vi "ParseSpeeds.vi"(8 "inputCluster":T1={"swerveModules"={"leftFront"={"driveCANID"=0.0, "angleCANID"=0, "canCoderCANID"=0.0, "moduleName"="", "driveMotorNeutralMode"=enum."EEPROMSetting", "driveCurrentLimitConfig"={"Enable?"=FALSE, "Current Limit"=0.0, "Threshold Current"=0.0, "Threshold Time"=0.0}, "driveFeedbackDevice"=0, "driveInitialSensorPosition"=0.0, "driveEnableVoltageComp"=FALSE, "driveVoltageComp"=0.0, "driveRampRate"=0.0, "angleCurrentLimit"=0.0, "angleSensorType"=enum."No Sensor", "angleMotorType"=enum."Brushed", "angleConversionFactor"=0.0, "anglePIDRamp"=0.0, "angleVoltageComp"=0.0, "angleIdleMode"=enum."Coast", "cancoderConfig"={"Sensor Initialization Strategy"=enum."Boot To Zero", "Absolute Sensor Range"=enum."Unsigned [0 to 360)", "Velocity Measurement Period"=0, "Velocity Measurement Window"=0, "Magnet Offset (Degrees)"=0.0, "Sensor Direction"=FALSE, "Sensor Coefficient"=0.0, "Unit String"="", "Sensor Time Base"=enum."Per100Ms_Legacy"}, "angleInitialSensorPosition"=0.0}, "rightFront"={"driveCANID"=0.0, "angleCANID"=0, "canCoderCANID"=0.0, "moduleName"="", "driveMotorNeutralMode"=enum."EEPROMSetting", "driveCurrentLimitConfig"={"Enable?"=FALSE, "Current Limit"=0.0, "Threshold Current"=0.0, "Threshold Time"=0.0}, "driveFeedbackDevice"=0, "driveInitialSensorPosition"=0.0, "driveEnableVoltageComp"=FALSE, "driveVoltageComp"=0.0, "driveRampRate"=0.0, "angleCurrentLimit"=0.0, "angleSensorType"=enum."No Sensor", "angleMotorType"=enum."Brushed", "angleConversionFactor"=0.0, "anglePIDRamp"=0.0, "angleVoltageComp"=0.0, "angleIdleMode"=enum."Coast", "cancoderConfig"={"Sensor Initialization Strategy"=enum."Boot To Zero", "Absolute Sensor Range"=enum."Unsigned [0 to 360)", "Velocity Measurement Period"=0, "Velocity Measurement Window"=0, "Magnet Offset (Degrees)"=0.0, "Sensor Direction"=FALSE, "Sensor Coefficient"=0.0, "Unit String"="", "Sensor Time Base"=enum."Per100Ms_Legacy"}, "angleInitialSensorPosition"=0.0}, "leftRear"={"driveCANID"=0.0, "angleCANID"=0, "canCoderCANID"=0.0, "moduleName"="", "driveMotorNeutralMode"=enum."EEPROMSetting", "driveCurrentLimitConfig"={"Enable?"=FALSE, "Current Limit"=0.0, "Threshold Current"=0.0, "Threshold Time"=0.0}, "driveFeedbackDevice"=0, "driveInitialSensorPosition"=0.0, "driveEnableVoltageComp"=FALSE, "driveVoltageComp"=0.0, "driveRampRate"=0.0, "angleCurrentLimit"=0.0, "angleSensorType"=enum."No Sensor", "angleMotorType"=enum."Brushed", "angleConversionFactor"=0.0, "anglePIDRamp"=0.0, "angleVoltageComp"=0.0, "angleIdleMode"=enum."Coast", "cancoderConfig"={"Sensor Initialization Strategy"=enum."Boot To Zero", "Absolute Sensor Range"=enum."Unsigned [0 to 360)", "Velocity Measurement Period"=0, "Velocity Measurement Window"=0, "Magnet Offset (Degrees)"=0.0, "Sensor Direction"=FALSE, "Sensor Coefficient"=0.0, "Unit String"="", "Sensor Time Base"=enum."Per100Ms_Legacy"}, "angleInitialSensorPosition"=0.0}, "rightRear"={"driveCANID"=0.0, "angleCANID"=0, "canCoderCANID"=0.0, "moduleName"="", "driveMotorNeutralMode"=enum."EEPROMSetting", "driveCurrentLimitConfig"={"Enable?"=FALSE, "Current Limit"=0.0, "Threshold Current"=0.0, "Threshold Time"=0.0}, "driveFeedbackDevice"=0, "driveInitialSensorPosition"=0.0, "driveEnableVoltageComp"=FALSE, "driveVoltageComp"=0.0, "driveRampRate"=0.0, "angleCurrentLimit"=0.0, "angleSensorType"=enum."No Sensor", "angleMotorType"=enum."Brushed", "angleConversionFactor"=0.0, "anglePIDRamp"=0.0, "angleVoltageComp"=0.0, "angleIdleMode"=enum."Coast", "cancoderConfig"={"Sensor Initialization Strategy"=enum."Boot To Zero", "Absolute Sensor Range"=enum."Unsigned [0 to 360)", "Velocity Measurement Period"=0, "Velocity Measurement Window"=0, "Magnet Offset (Degrees)"=0.0, "Sensor Direction"=FALSE, "Sensor Coefficient"=0.0, "Unit String"="", "Sensor Time Base"=enum."Per100Ms_Legacy"}, "angleInitialSensorPosition"=0.0}}, "offsets"={"leftFrontAngleOffset"=-143.789, "leftRearAngleOffset"=-94.834, "rightFrontAngleOffset"=55.1074, "rightRearAngleOffset"=42.8906}, "limits"={"maxVelocity"=0.0, "maxOverdriveVelocity"=0.0, "maxAcceleration"=0.0, "maxPickupVelocity"=0.0}, "speeds"={"intakeSuckSpeed"=0.0, "intakeSpitSpeed"=0.0, "indexerSuckSpeed"=0.0, "indexerSpitSpeed"=0.0, "indexerShootSpeed"=0.0, "indexerBumpBackSpeed"=0.0, "shooterSpinupSpeed"=0.0, "kickupSpinupSpeed"=0.0, "shooterLowShootSpeed"=0.0, "shooterHighShootSpeed"=0.0}, "positions"={"intakeStarting"=0.0, "intakeStow"=0.0, "intakeSuck"=0.0, "armPounce"=0.0, "armStow"=0.0, "armUp"=0.0, "winchPounce"=0.0, "winchOut"=0.0, "winchStow"=0.0, "intakeSpit"=0.0, "winchBarEngage"=0.0, "winchBottomClimb"=0.0, "hoodHighShoot"=0.0}, "inversions"={"rightShooter"=FALSE, "leftShooter"=FALSE}} {"swerveModules"."rightRear"."cancoderConfig"."Velocity Measurement Period" items=["Period_1ms"=1, "Period_2ms"=2, "Period_5ms"=5, "Period_10ms"=10, "Period_20ms"=20, "Period_25ms"=25, "Period_50ms"=50, "Period_100ms"=100]; "swerveModules"."rightRear"."cancoderConfig"."Sensor Coefficient" format="%#_9g"; "swerveModules"."rightRear"."driveFeedbackDevice" items=["Integrated Sensor"=1, "Sensor Sum (S0 + S1)"=9, "Sensor Difference (D0 - D1)"=10, "Remote Source 0"=11, "Remote Source 1"=12, "None"=14, "Software Emulated"=15]; "swerveModules"."leftRear"."cancoderConfig"."Velocity Measurement Period" items=["Period_1ms"=1, "Period_2ms"=2, "Period_5ms"=5, "Period_10ms"=10, "Period_20ms"=20, "Period_25ms"=25, "Period_50ms"=50, "Period_100ms"=100]; "swerveModules"."leftRear"."cancoderConfig"."Sensor Coefficient" format="%#_9g"; "swerveModules"."leftRear"."driveFeedbackDevice" items=["Integrated Sensor"=1, "Sensor Sum (S0 + S1)"=9, "Sensor Difference (D0 - D1)"=10, "Remote Source 0"=11, "Remote Source 1"=12, "None"=14, "Software Emulated"=15]; "swerveModules"."rightFront"."cancoderConfig"."Velocity Measurement Period" items=["Period_1ms"=1, "Period_2ms"=2, "Period_5ms"=5, "Period_10ms"=10, "Period_20ms"=20, "Period_25ms"=25, "Period_50ms"=50, "Period_100ms"=100]; "swerveModules"."rightFront"."cancoderConfig"."Sensor Coefficient" format="%#_9g"; "swerveModules"."rightFront"."driveFeedbackDevice" items=["Integrated Sensor"=1, "Sensor Sum (S0 + S1)"=9, "Sensor Difference (D0 - D1)"=10, "Remote Source 0"=11, "Remote Source 1"=12, "None"=14, "Software Emulated"=15]; "swerveModules"."leftFront"."cancoderConfig"."Velocity Measurement Period" items=["Period_1ms"=1, "Period_2ms"=2, "Period_5ms"=5, "Period_10ms"=10, "Period_20ms"=20, "Period_25ms"=25, "Period_50ms"=50, "Period_100ms"=100]; "swerveModules"."leftFront"."cancoderConfig"."Sensor Coefficient" format="%#_9g"; "swerveModules"."leftFront"."driveFeedbackDevice" items=["Integrated Sensor"=1, "Sensor Sum (S0 + S1)"=9, "Sensor Difference (D0 - D1)"=10, "Remote Source 0"=11, "Remote Source 1"=12, "None"=14, "Software Emulated"=15]}, 9 "configRef":T14) -> (2 "outputCluster":T1={"swerveModules"={"leftFront"={"driveCANID"=0.0, "angleCANID"=0, "canCoderCANID"=0.0, "moduleName"="", "driveMotorNeutralMode"=enum."EEPROMSetting", "driveCurrentLimitConfig"={"Enable?"=FALSE, "Current Limit"=0.0, "Threshold Current"=0.0, "Threshold Time"=0.0}, "driveFeedbackDevice"=0, "driveInitialSensorPosition"=0.0, "driveEnableVoltageComp"=FALSE, "driveVoltageComp"=0.0, "driveRampRate"=0.0, "angleCurrentLimit"=0.0, "angleSensorType"=enum."No Sensor", "angleMotorType"=enum."Brushed", "angleConversionFactor"=0.0, "anglePIDRamp"=0.0, "angleVoltageComp"=0.0, "angleIdleMode"=enum."Coast", "cancoderConfig"={"Sensor Initialization Strategy"=enum."Boot To Zero", "Absolute Sensor Range"=enum."Unsigned [0 to 360)", "Velocity Measurement Period"=0, "Velocity Measurement Window"=0, "Magnet Offset (Degrees)"=0.0, "Sensor Direction"=FALSE, "Sensor Coefficient"=0.0, "Unit String"="", "Sensor Time Base"=enum."Per100Ms_Legacy"}, "angleInitialSensorPosition"=0.0}, "rightFront"={"driveCANID"=0.0, "angleCANID"=0, "canCoderCANID"=0.0, "moduleName"="", "driveMotorNeutralMode"=enum."EEPROMSetting", "driveCurrentLimitConfig"={"Enable?"=FALSE, "Current Limit"=0.0, "Threshold Current"=0.0, "Threshold Time"=0.0}, "driveFeedbackDevice"=0, "driveInitialSensorPosition"=0.0, "driveEnableVoltageComp"=FALSE, "driveVoltageComp"=0.0, "driveRampRate"=0.0, "angleCurrentLimit"=0.0, "angleSensorType"=enum."No Sensor", "angleMotorType"=enum."Brushed", "angleConversionFactor"=0.0, "anglePIDRamp"=0.0, "angleVoltageComp"=0.0, "angleIdleMode"=enum."Coast", "cancoderConfig"={"Sensor Initialization Strategy"=enum."Boot To Zero", "Absolute Sensor Range"=enum."Unsigned [0 to 360)", "Velocity Measurement Period"=0, "Velocity Measurement Window"=0, "Magnet Offset (Degrees)"=0.0, "Sensor Direction"=FALSE, "Sensor Coefficient"=0.0, "Unit String"="", "Sensor Time Base"=enum."Per100Ms_Legacy"}, "angleInitialSensorPosition"=0.0}, "leftRear"={"driveCANID"=0.0, "angleCANID"=0, "canCoderCANID"=0.0, "moduleName"="", "driveMotorNeutralMode"=enum."EEPROMSetting", "driveCurrentLimitConfig"={"Enable?"=FALSE, "Current Limit"=0.0, "Threshold Current"=0.0, "Threshold Time"=0.0}, "driveFeedbackDevice"=0, "driveInitialSensorPosition"=0.0, "driveEnableVoltageComp"=FALSE, "driveVoltageComp"=0.0, "driveRampRate"=0.0, "angleCurrentLimit"=0.0, "angleSensorType"=enum."No Sensor", "angleMotorType"=enum."Brushed", "angleConversionFactor"=0.0, "anglePIDRamp"=0.0, "angleVoltageComp"=0.0, "angleIdleMode"=enum."Coast", "cancoderConfig"={"Sensor Initialization Strategy"=enum."Boot To Zero", "Absolute Sensor Range"=enum."Unsigned [0 to 360)", "Velocity Measurement Period"=0, "Velocity Measurement Window"=0, "Magnet Offset (Degrees)"=0.0, "Sensor Direction"=FALSE, "Sensor Coefficient"=0.0, "Unit String"="", "Sensor Time Base"=enum."Per100Ms_Legacy"}, "angleInitialSensorPosition"=0.0}, "rightRear"={"driveCANID"=0.0, "angleCANID"=0, "canCoderCANID"=0.0, "moduleName"="", "driveMotorNeutralMode"=enum."EEPROMSetting", "driveCurrentLimitConfig"={"Enable?"=FALSE, "Current Limit"=0.0, "Threshold Current"=0.0, "Threshold Time"=0.0}, "driveFeedbackDevice"=0, "driveInitialSensorPosition"=0.0, "driveEnableVoltageComp"=FALSE, "driveVoltageComp"=0.0, "driveRampRate"=0.0, "angleCurrentLimit"=0.0, "angleSensorType"=enum."No Sensor", "angleMotorType"=enum."Brushed", "angleConversionFactor"=0.0, "anglePIDRamp"=0.0, "angleVoltageComp"=0.0, "angleIdleMode"=enum."Coast", "cancoderConfig"={"Sensor Initialization Strategy"=enum."Boot To Zero", "Absolute Sensor Range"=enum."Unsigned [0 to 360)", "Velocity Measurement Period"=0, "Velocity Measurement Window"=0, "Magnet Offset (Degrees)"=0.0, "Sensor Direction"=FALSE, "Sensor Coefficient"=0.0, "Unit String"="", "Sensor Time Base"=enum."Per100Ms_Legacy"}, "angleInitialSensorPosition"=0.0}}, "offsets"={"leftFrontAngleOffset"=-143.789, "leftRearAngleOffset"=-94.834, "rightFrontAngleOffset"=55.1074, "rightRearAngleOffset"=42.8906}, "limits"={"maxVelocity"=0.0, "maxOverdriveVelocity"=0.0, "maxAcceleration"=0.0, "maxPickupVelocity"=0.0}, "speeds"={"intakeSuckSpeed"=0.0, "intakeSpitSpeed"=0.0, "indexerSuckSpeed"=0.0, "indexerSpitSpeed"=0.0, "indexerShootSpeed"=0.0, "indexerBumpBackSpeed"=0.0, "shooterSpinupSpeed"=0.0, "kickupSpinupSpeed"=0.0, "shooterLowShootSpeed"=0.0, "shooterHighShootSpeed"=0.0}, "positions"={"intakeStarting"=0.0, "intakeStow"=0.0, "intakeSuck"=0.0, "armPounce"=0.0, "armStow"=0.0, "armUp"=0.0, "winchPounce"=0.0, "winchOut"=0.0, "winchStow"=0.0, "intakeSpit"=0.0, "winchBarEngage"=0.0, "winchBottomClimb"=0.0, "hoodHighShoot"=0.0}, "inversions"={"rightShooter"=FALSE, "leftShooter"=FALSE}} {"swerveModules"."rightRear"."cancoderConfig"."Velocity Measurement Period" items=["Period_1ms"=1, "Period_2ms"=2, "Period_5ms"=5, "Period_10ms"=10, "Period_20ms"=20, "Period_25ms"=25, "Period_50ms"=50, "Period_100ms"=100]; "swerveModules"."rightRear"."cancoderConfig"."Sensor Coefficient" format="%#_9g"; "swerveModules"."rightRear"."driveFeedbackDevice" items=["Integrated Sensor"=1, "Sensor Sum (S0 + S1)"=9, "Sensor Difference (D0 - D1)"=10, "Remote Source 0"=11, "Remote Source 1"=12, "None"=14, "Software Emulated"=15]; "swerveModules"."leftRear"."cancoderConfig"."Velocity Measurement Period" items=["Period_1ms"=1, "Period_2ms"=2, "Period_5ms"=5, "Period_10ms"=10, "Period_20ms"=20, "Period_25ms"=25, "Period_50ms"=50, "Period_100ms"=100]; "swerveModules"."leftRear"."cancoderConfig"."Sensor Coefficient" format="%#_9g"; "swerveModules"."leftRear"."driveFeedbackDevice" items=["Integrated Sensor"=1, "Sensor Sum (S0 + S1)"=9, "Sensor Difference (D0 - D1)"=10, "Remote Source 0"=11, "Remote Source 1"=12, "None"=14, "Software Emulated"=15]; "swerveModules"."rightFront"."cancoderConfig"."Velocity Measurement Period" items=["Period_1ms"=1, "Period_2ms"=2, "Period_5ms"=5, "Period_10ms"=10, "Period_20ms"=20, "Period_25ms"=25, "Period_50ms"=50, "Period_100ms"=100]; "swerveModules"."rightFront"."cancoderConfig"."Sensor Coefficient" format="%#_9g"; "swerveModules"."rightFront"."driveFeedbackDevice" items=["Integrated Sensor"=1, "Sensor Sum (S0 + S1)"=9, "Sensor Difference (D0 - D1)"=10, "Remote Source 0"=11, "Remote Source 1"=12, "None"=14, "Software Emulated"=15]; "swerveModules"."leftFront"."cancoderConfig"."Velocity Measurement Period" items=["Period_1ms"=1, "Period_2ms"=2, "Period_5ms"=5, "Period_10ms"=10, "Period_20ms"=20, "Period_25ms"=25, "Period_50ms"=50, "Period_100ms"=100]; "swerveModules"."leftFront"."cancoderConfig"."Sensor Coefficient" format="%#_9g"; "swerveModules"."leftFront"."driveFeedbackDevice" items=["Integrated Sensor"=1, "Sensor Sum (S0 + S1)"=9, "Sensor Difference (D0 - D1)"=10, "Remote Source 0"=11, "Remote Source 1"=12, "None"=14, "Software Emulated"=15]}, 3 "configRefOut":T14)   [LabVIEW 2020]
uses:
  <vilib>/Utility/config.llb/Config Data RefNum.ctl
  PiConfig.ctl
  Swerve System/Swerve Module Parameters.ctl
  <vilib>/Rock Robotics/WPI/ThirdParty/Phoenix-LabVIEW/Motor Controller/Controls/CTRE_Phoenix_MotorControl_NeutralMode.ctl
  <vilib>/Rock Robotics/WPI/ThirdParty/Phoenix-LabVIEW/Motor Controller/Controls/CTRE_Phoenix_MotorControl_SupplyCurrentLimitConfiguration.ctl
  <vilib>/Rock Robotics/WPI/ThirdParty/Phoenix-LabVIEW/Motor Controller/Controls/CTRE_Phoenix_MotorControl_FeedbackDevice_TalonFX.ctl
  <vilib>/Rock Robotics/WPI/ThirdParty/REV Robotics/REVLib/Typedef/Spark MAX Sensor Type.ctl
  <vilib>/Rock Robotics/WPI/ThirdParty/REV Robotics/REVLib/Typedef/Spark MAX Motor Type.ctl
  <vilib>/Rock Robotics/WPI/ThirdParty/REV Robotics/REVLib/Typedef/Spark MAX Idle Mode.ctl
  <vilib>/Rock Robotics/WPI/ThirdParty/Phoenix-LabVIEW/CANCoder/Controls/CTRE_Phoenix_CANcoder_Configurables.ctl
  <vilib>/Rock Robotics/WPI/ThirdParty/Phoenix-LabVIEW/CANCoder/Controls/CTRE_Phoenix_CANcoder_SensorInitializationStrategy.ctl
  <vilib>/Rock Robotics/WPI/ThirdParty/Phoenix-LabVIEW/CANCoder/Controls/CTRE_Phoenix_CANcoder_AbsoluteSensorRange.ctl
  <vilib>/Rock Robotics/WPI/ThirdParty/Phoenix-LabVIEW/Motor Controller/Controls/CTRE_Phoenix_MotorControl_VelocityMeasurementPeriod.ctl
  <vilib>/Rock Robotics/WPI/ThirdParty/Phoenix-LabVIEW/CANCoder/Controls/CTRE_Phoenix_CANcoder_SensorTimeBase.ctl
  <vilib>/Utility/config.llb/Read Key (Double).vi
  <vilib>/Utility/config.llb/NI_LVConfig.lvlib
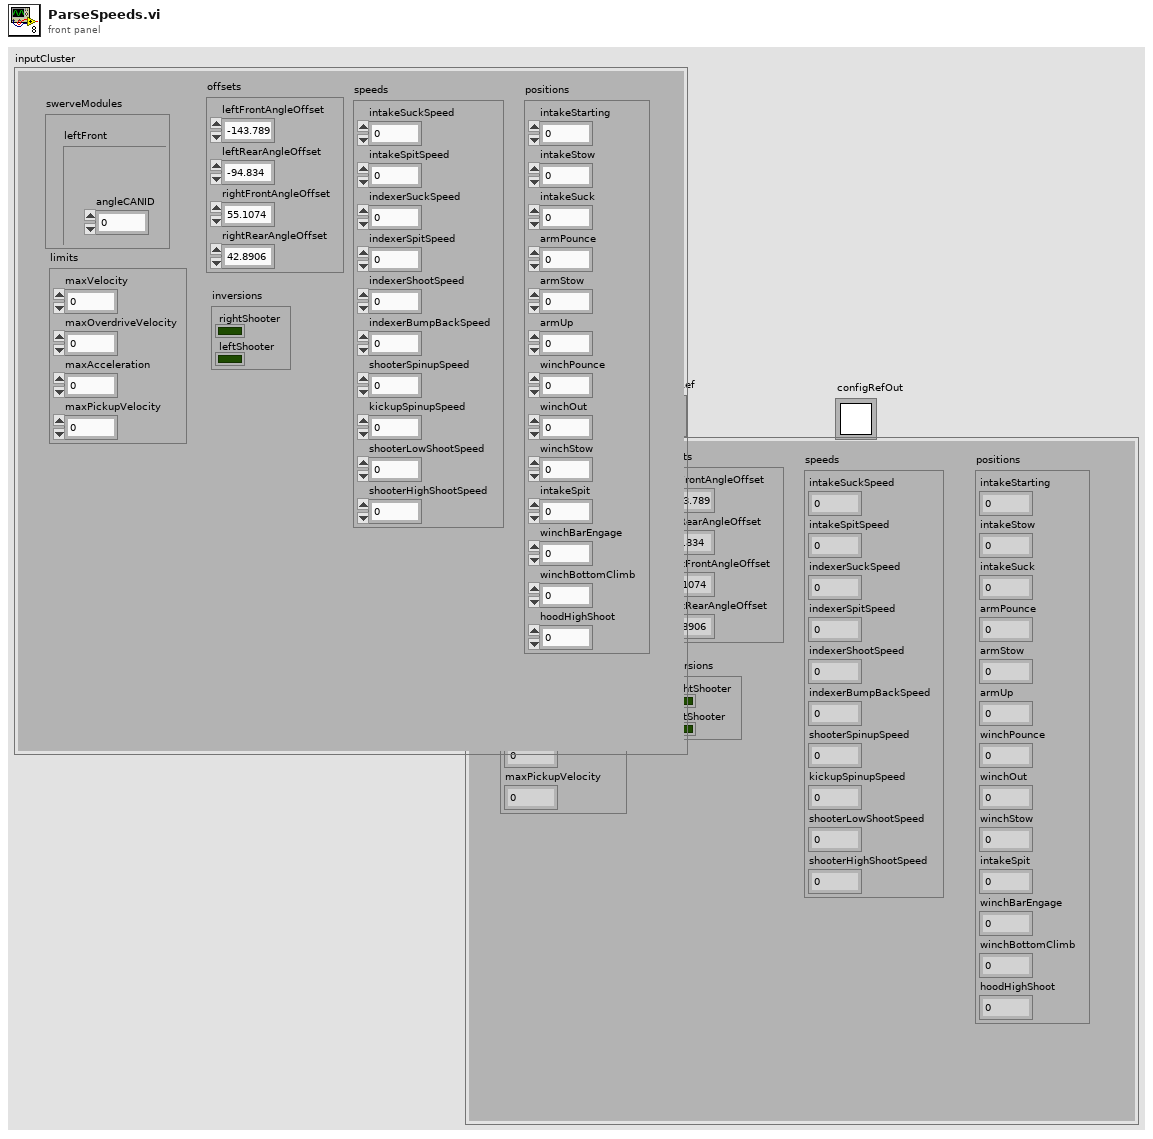
[diagram p1: front panel]
types:
  T1 = typedef "PiConfig.ctl" = cluster{"swerveModules":cluster{"leftFront":T2, "rightFront":T2, "leftRear":T2, "rightRear":T2}, "offsets":cluster{"leftFrontAngleOffset":dbl, "leftRearAngleOffset":dbl, "rightFrontAngleOffset":dbl, "rightRearAngleOffset":dbl}, "limits":cluster{"maxVelocity":dbl, "maxOverdriveVelocity":dbl, "maxAcceleration":dbl, "maxPickupVelocity":dbl}, "speeds":cluster{"intakeSuckSpeed":dbl, "intakeSpitSpeed":dbl, "indexerSuckSpeed":dbl, "indexerSpitSpeed":dbl, "indexerShootSpeed":dbl, "indexerBumpBackSpeed":dbl, "shooterSpinupSpeed":dbl, "kickupSpinupSpeed":dbl, "shooterLowShootSpeed":dbl, "shooterHighShootSpeed":dbl}, "positions":cluster{"intakeStarting":dbl, "intakeStow":dbl, "intakeSuck":dbl, "armPounce":dbl, "armStow":dbl, "armUp":dbl, "winchPounce":dbl, "winchOut":dbl, "winchStow":dbl, "intakeSpit":dbl, "winchBarEngage":dbl, "winchBottomClimb":dbl, "hoodHighShoot":dbl}, "inversions":cluster{"rightShooter":bool, "leftShooter":bool}}
  T2 = typedef "Swerve Module Parameters.ctl" = cluster{"driveCANID":dbl, "angleCANID":i32, "canCoderCANID":dbl, "moduleName":string, "driveMotorNeutralMode":T3, "driveCurrentLimitConfig":T4, "driveFeedbackDevice":T5, "driveInitialSensorPosition":dbl, "driveEnableVoltageComp":bool, "driveVoltageComp":dbl, "driveRampRate":dbl, "angleCurrentLimit":dbl, "angleSensorType":T6, "angleMotorType":T7, "angleConversionFactor":dbl, "anglePIDRamp":dbl, "angleVoltageComp":dbl, "angleIdleMode":T8, "cancoderConfig":T9, "angleInitialSensorPosition":dbl}
  T3 = typedef "CTRE_Phoenix_MotorControl_NeutralMode.ctl" = enum8{"EEPROMSetting", "Override to Coast", "Override to Brake"}
  T4 = typedef "CTRE_Phoenix_MotorControl_SupplyCurrentLimitConfiguration.ctl" = cluster{"Enable?":bool, "Current Limit":dbl, "Threshold Current":dbl, "Threshold Time":dbl}
  T5 = typedef "CTRE_Phoenix_MotorControl_FeedbackDevice_TalonFX.ctl" = i8
  T6 = typedef "Spark MAX Sensor Type.ctl" = enum16{"No Sensor", "Hall Sensor", "Encoder", "-Not Available-", "Analog", "Alternate Encoder"}
  T7 = typedef "Spark MAX Motor Type.ctl" = enum16{"Brushed", "Brushless"}
  T8 = typedef "Spark MAX Idle Mode.ctl" = enum16{"Coast", "Brake"}
  T9 = typedef "CTRE_Phoenix_CANcoder_Configurables.ctl" = cluster{"Sensor Initialization Strategy":T10, "Absolute Sensor Range":T11, "Velocity Measurement Period":T12, "Velocity Measurement Window":i32, "Magnet Offset (Degrees)":dbl, "Sensor Direction":bool, "Sensor Coefficient":dbl, "Unit String":string, "Sensor Time Base":T13}
  T10 = typedef "CTRE_Phoenix_CANcoder_SensorInitializationStrategy.ctl" = enum16{"Boot To Zero", "Boot To Absolute Position"}
  T11 = typedef "CTRE_Phoenix_CANcoder_AbsoluteSensorRange.ctl" = enum16{"Unsigned [0 to 360)", "Signed [-180 to +180)"}
  T12 = typedef "CTRE_Phoenix_MotorControl_VelocityMeasurementPeriod.ctl" = u16
  T13 = typedef "CTRE_Phoenix_CANcoder_SensorTimeBase.ctl" = enum16{"Per100Ms_Legacy", "PerSecond", "PerMinute"}
  T14 = typedef "NI_LVConfig.lvlib/Config Data RefNum.ctl" = refnum<k1>
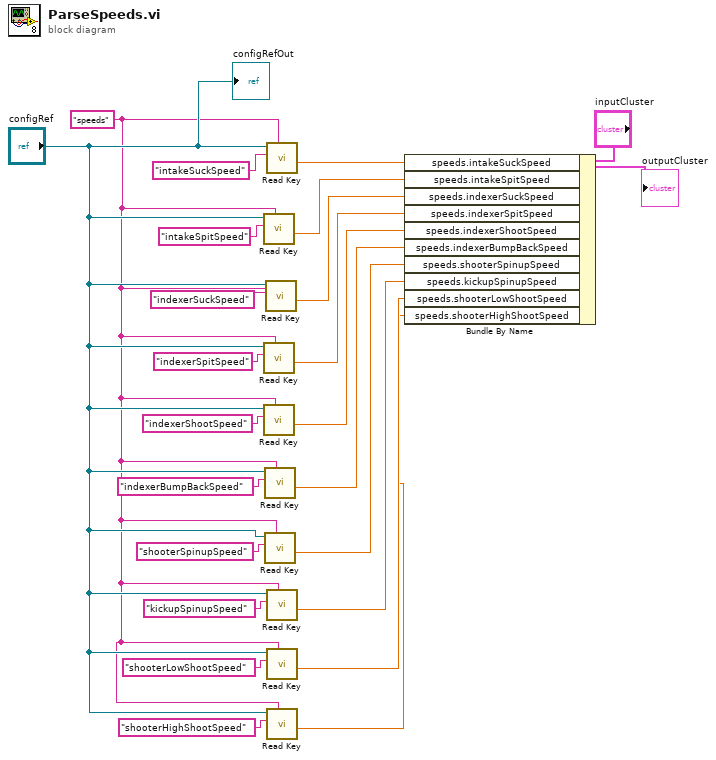
[diagram p0: block diagram]
diagram:
  w3 = "speeds" ("section")
  n1 = call-poly <vilib>:"Read Key.vi"("section"=w3, "key"="intakeSpitSpeed", "refnum"="configRef") -> ("value"=w14:dbl)  [unwired: 5 in, 3 out]
  n2 = call-poly <vilib>:"Read Key.vi"("section"=w3, "key"="indexerSpitSpeed", "refnum"="configRef") -> ("value"=w12:dbl)  [unwired: 5 in, 3 out]
  n3 = call-poly <vilib>:"Read Key.vi"("section"=w3, "key"="indexerShootSpeed", "refnum"="configRef") -> ("value"=w11:dbl)  [unwired: 5 in, 3 out]
  n4 = call-poly <vilib>:"Read Key.vi"("section"=w3, "key"="indexerBumpBackSpeed", "refnum"="configRef") -> ("value"=w10:dbl)  [unwired: 5 in, 3 out]
  n5 = call-poly <vilib>:"Read Key.vi"("section"=w3, "key"="shooterSpinupSpeed", "refnum"="configRef") -> ("value"=w9:dbl)  [unwired: 5 in, 3 out]
  n6 = call-poly <vilib>:"Read Key.vi"("section"=w3, "key"="indexerSuckSpeed", "refnum"="configRef") -> ("value"=w13:dbl)  [unwired: 5 in, 3 out]
  n7 = call-poly <vilib>:"Read Key.vi"("section"=w3, "key"="intakeSuckSpeed", "refnum"="configRef") -> ("value"=w20:dbl)  [unwired: 5 in, 3 out]
  n8 = call-poly <vilib>:"Read Key.vi"("section"=w3, "key"="kickupSpinupSpeed", "refnum"="configRef") -> ("value"=w7:dbl)  [unwired: 5 in, 3 out]
  n9 = call-poly <vilib>:"Read Key.vi"("section"=w3, "key"="shooterLowShootSpeed", "refnum"="configRef") -> ("value"=w2:dbl)  [unwired: 5 in, 3 out]
  n10 = call-poly <vilib>:"Read Key.vi"("section"=w3, "key"="shooterHighShootSpeed", "refnum"="configRef") -> ("value"=w1:dbl)  [unwired: 5 in, 3 out]
  n11 = Bundle By Name(cluster="inputCluster", "speeds.intakeSuckSpeed"=w20, "speeds.intakeSpitSpeed"=w14, "speeds.indexerSuckSpeed"=w13, "speeds.indexerSpitSpeed"=w12, "speeds.indexerShootSpeed"=w11, "speeds.indexerBumpBackSpeed"=w10, "speeds.shooterSpinupSpeed"=w9, "speeds.kickupSpinupSpeed"=w7, "speeds.shooterLowShootSpeed"=w2, "speeds.shooterHighShootSpeed"=w1) -> (→"outputCluster":T1)
  "configRefOut" <- "configRef"
